vi "Read Value.vi"(11 "Option in":refnum<class "Option.lvclass">) -> (1 "Set":bool, 2 "Value":string, 3 "Option out":refnum<class "Option.lvclass">)   [LabVIEW 2011, in "Option Parser.lvlib" / "Option.lvclass"]
uses:
  Option.lvclass
  Option.lvclass/Option.ctl
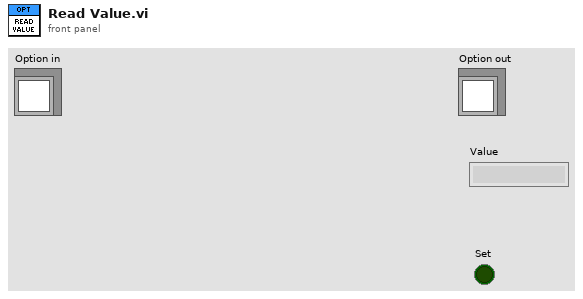
[diagram p1: front panel]
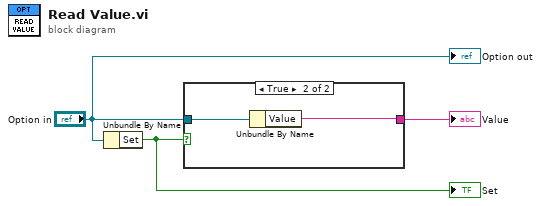
[diagram p0: block diagram]
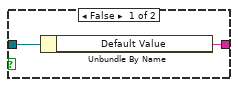
[diagram p2: hidden frame]
diagram:
  n1 = Unbundle By Name("Option in") -> ("Set"=w3:bool)
  "Set" <- w3
  n2 = case shown="True" w3 {
    tunnel: "Option in" -> [w5 w7]
    tunnel: [w4 w6] -> w1
    frame False {
      n3 = Unbundle By Name(w5) -> ("Default Value"=w4:string)
    }
    frame True {
      n4 = Unbundle By Name(w7) -> ("Value"=w6:string)
    }
  }
  "Value" <- w1
  "Option out" <- "Option in"
